vi "DefinePrecidence.vi"(1 "regular expression":string="[+-*/]", 2 "Script in":string) -> (0 "Script out":string)   [LabVIEW 2014]
panel:
  out "Array 2":string[][](array[string])
  out "Array":i32[][](array[numeric])
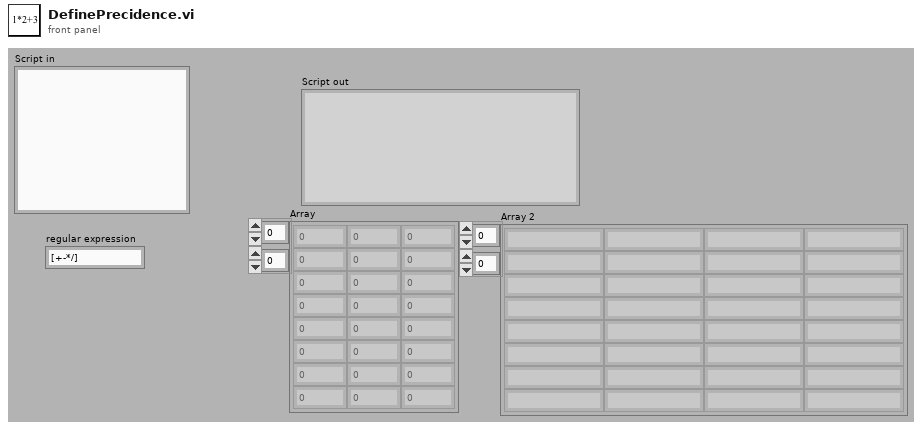
[diagram p1: front panel]
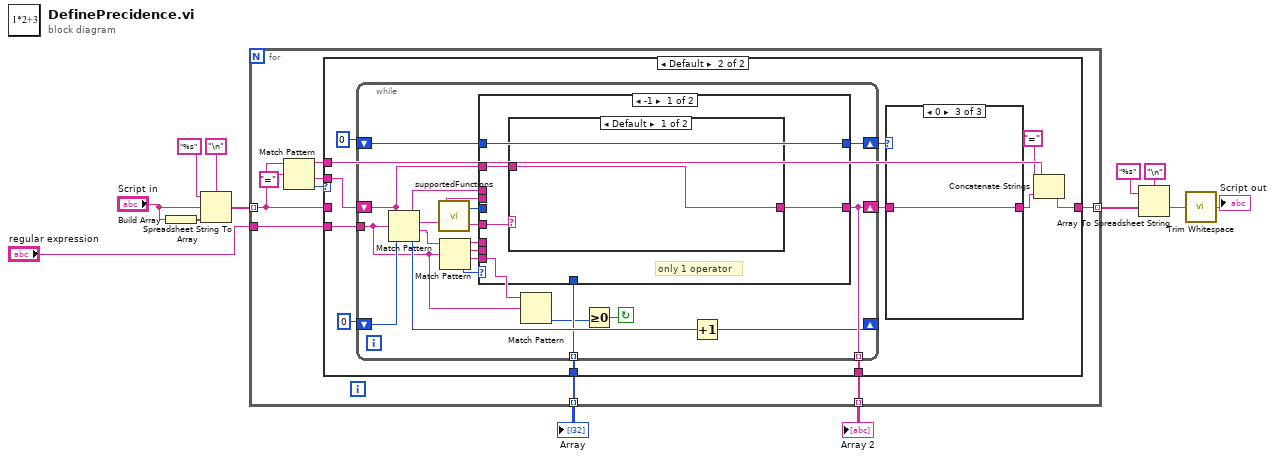
[diagram p0: block diagram]
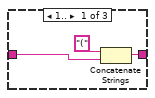
[diagram p3: hidden frame]
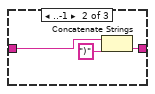
[diagram p4: hidden frame]
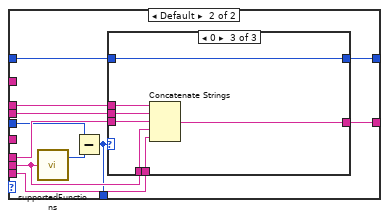
[diagram p6: hidden frame]
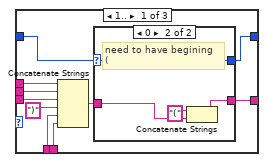
[diagram p7: hidden frame]
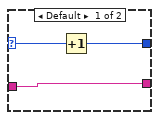
[diagram p8: hidden frame]
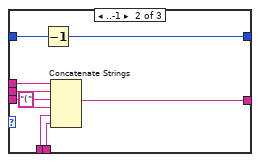
[diagram p9: hidden frame]
diagram:
  n1 = Build Array("Script in") -> (w13:string[])
  n2 = Spreadsheet String To Array(delimiter (Tab)="\n", format string="%s", spreadsheet string="Script in", array type (2D Dbl)=w13) -> (array=w10:string[])
  n3 = for {
    tunnel: w10 -> [w21] mode=indexing
    tunnel: "regular expression" -> [w22]
    tunnel: [w18] -> w7 mode=indexing
    tunnel: [w17] -> w4 mode=indexing
    tunnel: [w16] -> w2 mode=indexing
    n4 = Match Pattern(string=w21, regular expression="=") -> (before substring=w14:string, after substring=w15:string, offset past match=w19:i32)  [unwired: 1 in, 1 out]
    n5 = case shown="Default" w19 {
      tunnel: w22 -> [_ w35]
      tunnel: w21 -> [w23 _]
      tunnel: [w23 w24] -> w18
      tunnel: [_ w30] -> w17
      tunnel: [_ w29] -> w16
      tunnel: w15 -> [_ w28]
      tunnel: w14 -> [_ w26]
      frame -1 {
        # "no formula"
      }
      frame Default {
        n6 = while {
          tunnel: w35 -> [w49]
          shift-right: [w45] -> w31
          shift-left: w28 -> [w46]
          shift-right: [w44] -> _
          shift-left: 0 -> [w56]
          shift-right: [w53] -> w32
          shift-left: 0 -> [w54]
          tunnel: [w51] -> w30 mode=indexing
          tunnel: [w45] -> w29 mode=indexing
          stop <- w55 continue-if-true
          n7 = Match Pattern(string=w46, regular expression=w49, offset (0)=w56) -> (before substring=w61:string, match substring=w60:string, after substring=w62:string, offset past match=w52:i32)
          n8 = call <userlib>:"supportedFunctions.vi"("String"=w60) -> ("regular expression"=w43:string, "Priority"=w57:i32)
          n9 = Match Pattern(string=w62, regular expression=w49) -> (before substring=w59:string, match substring=w58:string, after substring=w50:string, offset past match=w47:i32)  [unwired: 1 in]
          n10 = case shown="-1" w47 {
            tunnel: [w64 w79] -> w45
            tunnel: w61 -> [_ w78]
            tunnel: w60 -> [_ w77]
            tunnel: w59 -> [_ w76]
            tunnel: w58 -> [_ w75]
            tunnel: w57 -> [_ w74]
            tunnel: w54 -> [w66 w72]
            tunnel: [w66 w71] -> w53
            tunnel: [_ w70] -> w51
            tunnel: w50 -> [_ w69]
            tunnel: w46 -> [w63 _]
            tunnel: w43 -> [w65 _]
            frame -1 {
              # "only 1 operator"
              n11 = case shown="Default" w65 {
                tunnel: [w67 w68] -> w64
                tunnel: w63 -> [w67 w68]
                frame Default {
                }
                frame "NOT" {
                }
              }
            }
            frame Default {
              n12 = call <userlib>:"supportedFunctions.vi"("String"=w75) -> ("Priority"=w73:i32)  [unwired: 1 out]
              n13 = Subtract(x=w74, y=w73) -> (x-y=w70:i32)
              n14 = case shown="0" w70 {
                tunnel: [w82 w105 w112] -> w79
                tunnel: w78 -> [w89 w104 w111]
                tunnel: w77 -> [w88 w103 w110]
                tunnel: w76 -> [w87 w99 w109]
                tunnel: w75 -> [w85 w102 w108]
                tunnel: w69 -> [w84 w101 w107]
                tunnel: w72 -> [w83 w98 w106]
                tunnel: [w80 w97 w106] -> w71
                frame 1.. {
                  n15 = Concatenate Strings(w89, w88, w87, ")" ("string"), w85, w84) -> (w81:string)
                  n16 = case shown="0" w83 {
                    selector: w83 -> [w91 w94]
                    tunnel: [w92 w95] -> w82
                    tunnel: w81 -> [w92 w93]
                    tunnel: [w90 w94] -> w80
                    frame Default {
                      n17 = Increment(x=w91) -> (x+1=w90:i32)
                    }
                    frame 0 {
                      # "need to have begining\n("
                      n18 = Concatenate Strings("(" ("regular expression"), w93) -> (w95:string)
                    }
                  }
                }
                frame ..-1 {
                  n19 = Decrement(x=w98) -> (x-1=w97:i32)
                  n20 = Concatenate Strings(w104, w103, "(" ("string"), w99, w102, w101) -> (w105:string)
                }
                frame 0 {
                  n21 = Concatenate Strings(w111, w110, w109, w108, w107) -> (w112:string)
                }
              }
            }
          }
          n22 = Match Pattern(string=w50, regular expression=w49) -> (offset past match=w48:i32)  [unwired: 1 in, 3 out]
          n23 = Greater Or Equal To 0?(x=w48) -> (x >= 0?=w55:bool)
          n24 = Increment(x=w52) -> (x+1=w44:i32)
        }
        n25 = case shown="0" w32 {
          tunnel: [w37 w41 w42] -> w27
          tunnel: w31 -> [w36 w40 w42]
          frame 1.. {
            n26 = Concatenate Strings("(" ("regular expression"), w36) -> (w37:string)
          }
          frame ..-1 {
            n27 = Concatenate Strings(w40, ")" ("regular expression")) -> (w41:string)
          }
          frame 0 {
          }
        }
        n28 = Concatenate Strings(w26, "=" ("regular expression"), w27) -> (w24:string)
      }
    }
  }
  "Array" <- w4
  "Array 2" <- w2
  n29 = Array To Spreadsheet String(delimiter (Tab)="\n", array=w7, 3:"%s" ("format string")) -> (spreadsheet string=w8:string)
  n30 = call <vilib>:"Trim Whitespace.vi"("string"=w8) -> ("trimmed string"=→"Script out":string)  [unwired: 1 in]
